vi "SDG60ReadArbitraryWFMQ.vi"(4 "Timeout (40000 ms)":u32=40000, 8 "error in (no error)":errorcluster, 11 "VISA resource name":refnum<visa-resource-name>="USB0::0xF4EC::0x1101::SDG6XEBC5R0119::INSTR") -> (0 "error out":errorcluster, 3 "VISA resource name out":refnum<visa-resource-name>)   [LabVIEW 2018]
doc: "Creates and saves an arbitrary waveform in edit memory. \n\n<B>Note:</B>\n\nCreates an arbitrary waveform in edit memory and because of this, the waveform will remain stored on the instrument until deleted. If any sensitive information is contained in the arbitrary waveform, it is recommended that the waveform be deleted when finished."
panel:
  out "String":string
  in  "WFM Name":string="ARB1"
  # "No dots in the file name!"
  # "Will not be able to read large files WFM/Length,\nbut can tell they exist on device"
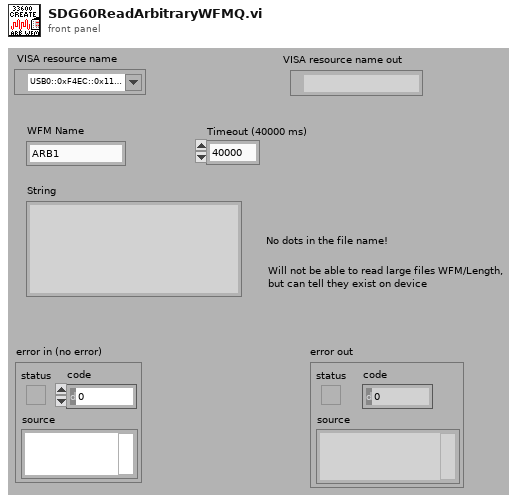
[diagram p1: front panel]
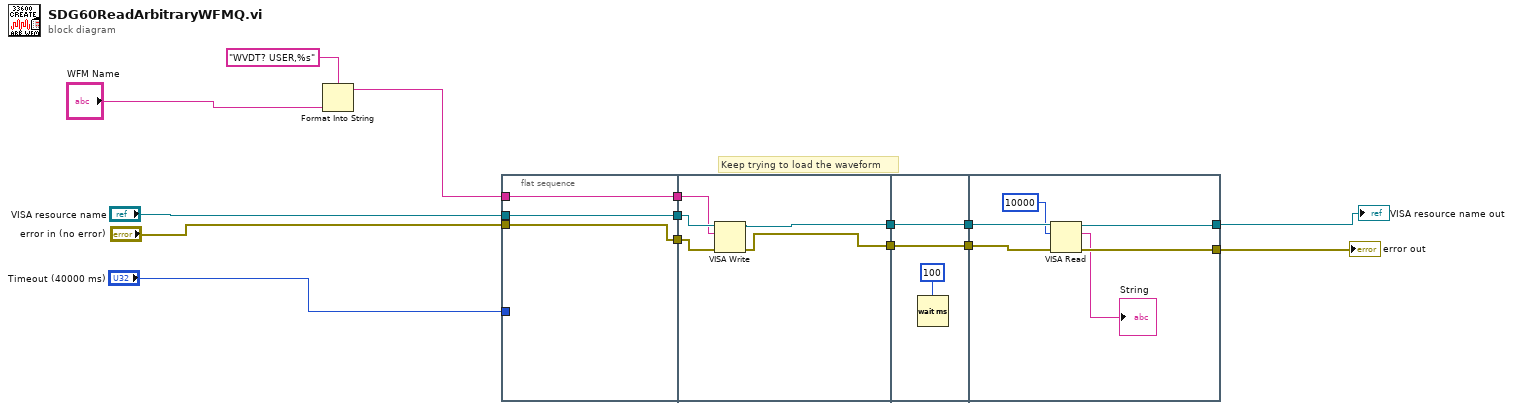
[diagram p0: block diagram]
diagram:
  # "Keep trying to load the waveform"
  n1 = Format Into String(format string="WVDT? USER,%s", "WFM Name") -> (resulting string=w10:string)  [unwired: 2 in, 1 out]
  n2 = flat-sequence {
    tunnel: [w16] -> w9
    tunnel: [w17] -> w8
    tunnel: w10 -> [w18]
    tunnel: [w18] -> w7
    tunnel: "Timeout (40000 ms)" -> [_]
    tunnel: "VISA resource name" -> [w16]
    tunnel: "error in (no error)" -> [w17]
    tunnel: w9 -> [w22]
    tunnel: w8 -> [w23]
    tunnel: w7 -> [w21]
    tunnel: [w19] -> w6
    tunnel: [w20] -> w5
    tunnel: w6 -> [w26]
    tunnel: [w26] -> w4
    tunnel: w5 -> [w25]
    tunnel: [w25] -> w3
    tunnel: [w31] -> w12
    tunnel: w4 -> [w30]
    tunnel: w3 -> [w32]
    tunnel: [w29] -> w1
    frame #0 {
    }
    frame #1 {
      n3 = VISA Write(VISA resource name=w22, write buffer=w21, error in (no error)=w23) -> (VISA resource name out=w20:refnum<visa-resource-name>, error out=w19:errorcluster)  [unwired: 1 out]
    }
    frame #2 {
      n4 = Wait (ms)(milliseconds to wait=100 ("x")) -> ()  [unwired: 1 out]
    }
    frame #3 {
      n5 = VISA Read(VISA resource name=w32, byte count=10000 ("x"), error in (no error)=w30) -> (VISA resource name out=w31:refnum<visa-resource-name>, read buffer=→"String":string, error out=w29:errorcluster)  [unwired: 1 out]
    }
  }
  "error out" <- w1
  "VISA resource name out" <- w12
